vi "ParseHeaders.vi"(0 "headers in":string, 11 "error in":errorcluster) -> (4 "status":u8, 6 "headers out":variant, 15 "error out":errorcluster)   [LabVIEW 2017, in "LabVIEWHTTPClient.lvlib"]
uses:
  <vilib>/httpClient/LabVIEWHTTPClient.lvlib
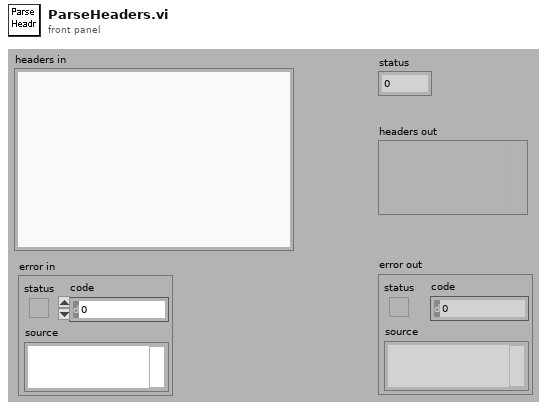
[diagram p1: front panel]
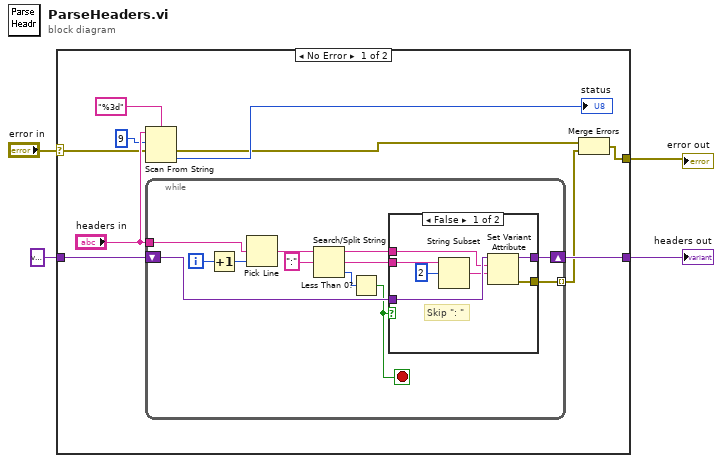
[diagram p0: block diagram]
diagram:
  n1 = case shown="No Error" "error in" {
    selector: "error in" -> [w9 w36]
    tunnel: [w14 w35] -> w4
    tunnel: [w5 w36] -> w1
    tunnel: variant ("variant") -> [w8 w35]
    frame No Error {
      n2 = Scan From String(format string="%3d", input string="headers in", initial scan location=u32 9, error in=w9) -> (error out=w6:errorcluster, output 1=→"status":u8)  [unwired: 1 in, 2 out]
      n3 = while {
        tunnel: "headers in" -> [w25]
        shift-right: [w24] -> w14
        shift-left: w8 -> [w26]
        tunnel: [w15] -> w7 mode=indexing
        i -> [w23]
        stop <- w16 stop-if-true
        n4 = Increment(x=w23) -> (x+1=w22:i32)
        n5 = Pick Line(multi-line string=w25, line index=w22) -> (output string=w20:string)  [unwired: 1 in]
        n6 = Search/Split String(string=w20, search string/char (-)=":") -> (substring before match=w17:string, match + rest of string=w18:string, offset of match=w21:i32)  [unwired: 1 in]
        n7 = Less Than 0?(x=w21) -> (x < 0?=w16:bool)
        n8 = case shown="False" w16 {
          tunnel: w26 -> [w33 w34]
          tunnel: [w32 w34] -> w24
          tunnel: w18 -> [w31 _]
          tunnel: w17 -> [w29 _]
          tunnel: [w27 _] -> w15
          frame False {
            # "Skip \": \""
            n9 = String Subset(string=w31, offset (0)=2) -> (substring=w28:string)  [unwired: 1 in]
            n10 = Set Variant Attribute(Variant=w33, name=w29, value=w28) -> (Variant out=w32:variant, error out=w27:errorcluster)  [unwired: 1 in, 1 out]
          }
          frame True {
          }
        }
      }
      n11 = Merge Errors(w6, w7) -> (w5:errorcluster)
    }
    frame Error {
    }
  }
  "headers out" <- w4
  "error out" <- w1
